vi "ComputeCOM.vi"(3 "Image":T1) -> (1 "Cluster 2":cluster{"comX":sgl, "comY":sgl})   [LabVIEW 2011]
uses:
  <vilib>/vision/Image Controls.llb/IMAQ Image.ctl
  cudatrack-debug.dll
panel:
  out "Numeric Indicator":dbl
  in  "comX":sgl
  in  "comY":sgl
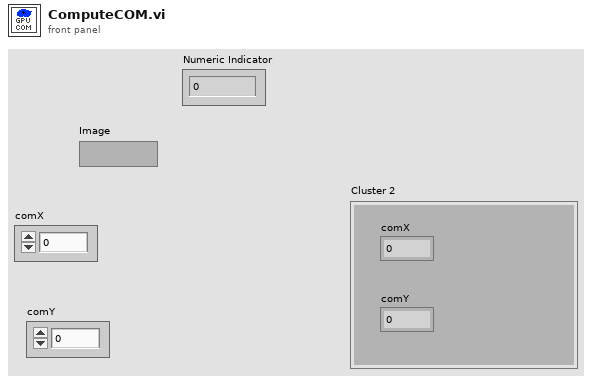
[diagram p1: front panel]
types:
  T1 = typedef "IMAQ Image.ctl" = refnum<image>
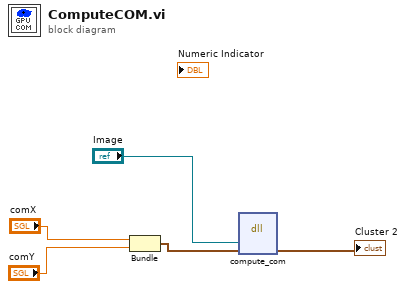
[diagram p0: block diagram]
diagram:
  n1 = Bundle("comX"="comX", "comY"="comY") -> (w3:cluster{"comX":sgl, "comY":sgl})  [unwired: 1 in]
  n2 = dll-call lib="D:/jcnossen1/cudaqi-tracker/cudaqi/cudatrack-debug.dll" fn="compute_com"("image"="Image", "position"=w3) -> ("position"=→"Cluster 2":cluster{"comX":sgl, "comY":sgl})  [unwired: 5 in, 2 out]
